vi "Remove Duplicates.vi"(3 "Array In":string[](array[string])) -> (1 "Array Out":string[](array[string]))   [LabVIEW 2019]
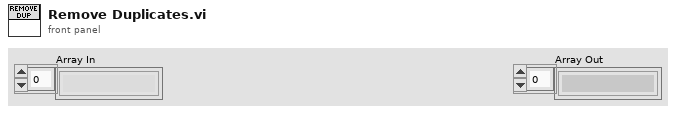
[diagram p1: front panel]
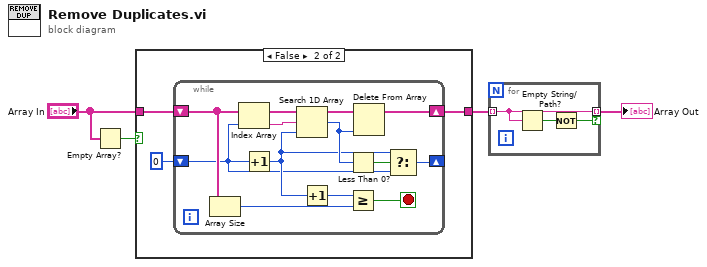
[diagram p0: block diagram]
diagram:
  n1 = Empty Array?(array="Array In") -> (empty?=w3:bool)
  n2 = case shown="False" w3 {
    tunnel: "Array In" -> [w5 w7]
    tunnel: [w5 w6] -> w2
    frame True {
    }
    frame False {
      n3 = while {
        shift-right: [w15] -> w6
        shift-left: w7 -> [w14]
        shift-right: [w19] -> _
        shift-left: 0 ("index") -> [w9]
        stop <- w16 stop-if-true
        n4 = Array Size(array=w14) -> (size(s)=w17:i32)
        n5 = Index Array(array=w14, index=w9) -> (element=w13:string)
        n6 = Increment(x=w9) -> (x+1=w10:i32)
        n7 = Search 1D Array(1D array=w14, element=w13, start index (0)=w10) -> (index of element=w12:i32)
        n8 = Increment(x=w10) -> (x+1=w18:i32)
        n9 = Less Than 0?(x=w12) -> (x < 0?=w11:bool)
        n10 = Greater Or Equal?(x=w18, y=w17) -> (x >= y?=w16:bool)
        n11 = Delete From Array(array=w14, index=w12) -> (array with subset deleted=w15:string[])  [unwired: 1 in, 1 out]
        n12 = Select(t=w10, s=w11, f=w9) -> (s? t:f=w19:i32)
      }
    }
  }
  n13 = for {
    tunnel: w2 -> [w22] mode=indexing
    tunnel: [w22] -> w1 mode=indexing if=w20
    n14 = Empty String/Path?(string/path=w22) -> (empty?=w21:bool)
    n15 = Not(x=w21) -> (.not. x?=w20:bool)
  }
  "Array Out" <- w1
